vi "Filter Changed DTCs.vi"(9 "Time Stamp":timestamp, 10 "Previous DTCs":T1(array[cluster]) {"Add Data" format="%.0x"; "Status" format="%.0x"; "DTC" format="%.0x"}, 11 "DTCs":T1(array[cluster]) {"Add Data" format="%.0x"; "Status" format="%.0x"; "DTC" format="%.0x"}) -> (3 "Changed DTCs":T2[](array[typedef]))   [LabVIEW 2015, in "Diagnostics Addon Engine.lvlib"]
uses:
  Diagnostics Addon Engine.lvlib
  Shared/Types/DTC.Info.ctl
  Shared/Diagnostics Addon Shared.lvlib
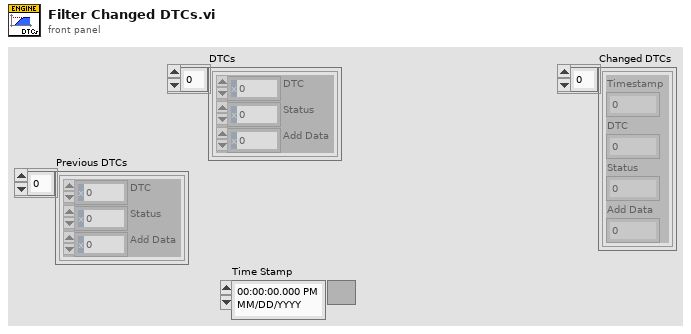
[diagram p1: front panel]
types:
  T1 = cluster{"DTC":u32, "Status":u32, "Add Data":u32}[]
  T2 = typedef "Diagnostics Addon Shared.lvlib/DTC.Info.ctl" = cluster{"Timestamp":dbl, "DTC":dbl, "Status":dbl, "Add Data":dbl}
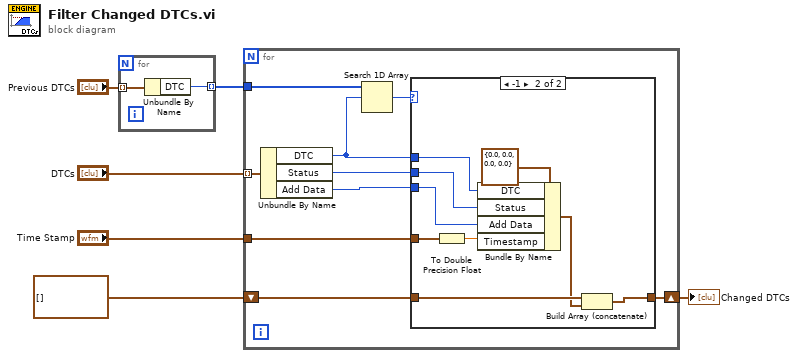
[diagram p0: block diagram]
diagram:
  n1 = for {
    tunnel: "Previous DTCs" -> [w8] mode=indexing
    tunnel: [w7] -> w6 mode=indexing
    n2 = Unbundle By Name(w8) -> ("DTC"=w7:u32)
  }
  n3 = for {
    tunnel: "DTCs" -> [w15] mode=indexing
    tunnel: w6 -> [w17]
    shift-right: [w13] -> w3
    shift-left: T2[] [] -> [w14]
    tunnel: "Time Stamp" -> [w12]
    n4 = Unbundle By Name(w15) -> ("DTC"=w10:u32, "Status"=w11:u32, "Add Data"=w9:u32)
    n5 = Search 1D Array(1D array=w17, element=w10) -> (index of element=w16:i32)  [unwired: 1 in]
    n6 = case shown="-1" w16 {
      tunnel: w14 -> [w18 w27]
      tunnel: [w18 w26] -> w13
      tunnel: w12 -> [_ w21]
      tunnel: w11 -> [_ w24]
      tunnel: w10 -> [_ w23]
      tunnel: w9 -> [_ w22]
      frame Default {
      }
      frame -1 {
        n7 = To Double Precision Float(number=w21) -> (double precision float=w20:dbl)
        n8 = Bundle By Name(cluster=T2 {"Timestamp"=0.0, "DTC"=0.0, "Status"=0.0, "Add Data"=0.0} ("Diagnostic Trouble Code"), "DTC"=w23, "Status"=w24, "Add Data"=w22, "Timestamp"=w20) -> (w19:T2)
        n9 = Build Array (concatenate)(w27, w19) -> (w26:T2[])
      }
    }
  }
  "Changed DTCs" <- w3
